vi "AvisoSectorConvert.vi"(7 "output cluster":T1={"Axis scaling Params"={"X right"=0.0, "X left"=0.0, "Y low"=0.0, "Y high"=0.0}, "x scaled"=[], "y scaled"=[], "scales"={"inc x (mm)"=0.0, "inc y (mm)"=0.0}, [], "pixels in x"=256, "pixels in y"=1000}, 10 "Log Lookup":sgl[](array[numeric]), 11 "Raw In":dbl[][](array[numeric])) -> (3 "Sector out":dbl[][](array[numeric]))   [LabVIEW 2022 SP3]
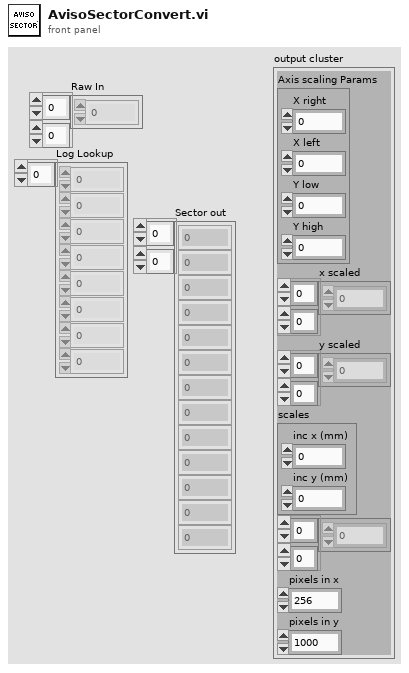
[diagram p1: front panel]
types:
  T1 = cluster{"Axis scaling Params":cluster{"X right":dbl, "X left":dbl, "Y low":dbl, "Y high":dbl}, "x scaled":dbl[][], "y scaled":dbl[][], "scales":cluster{"inc x (mm)":dbl, "inc y (mm)":dbl}, dbl[][], "pixels in x":i16, "pixels in y":i16}
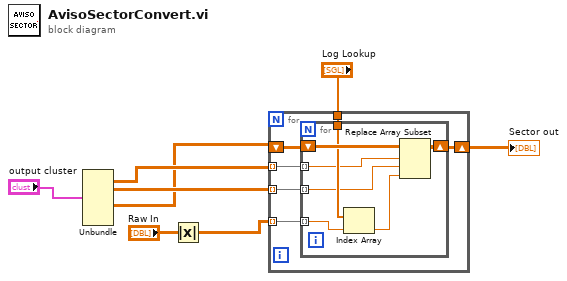
[diagram p0: block diagram]
diagram:
  n1 = Unbundle("output cluster") -> ("x scaled"=w5:dbl[][], "y scaled"=w6:dbl[][], w3:dbl[][])  [unwired: 4 out]
  n2 = Absolute Value(x="Raw In") -> (abs(x)=w4:dbl[][])
  n3 = for {
    tunnel: w4 -> [w14] mode=indexing
    shift-right: [w12] -> w1
    shift-left: w3 -> [w13]
    tunnel: w5 -> [w11] mode=indexing
    tunnel: w6 -> [w10] mode=indexing
    tunnel: "Log Lookup" -> [w9]
    n4 = for {
      tunnel: w14 -> [w19] mode=indexing
      shift-right: [w20] -> w12
      shift-left: w13 -> [w21]
      tunnel: w11 -> [w16] mode=indexing
      tunnel: w10 -> [w15] mode=indexing
      tunnel: w9 -> [w17]
      n5 = Index Array(array=w17, index=w19) -> (element=w18:sgl)
      n6 = Replace Array Subset(array=w21, new element=w18, index (row)=w16, index (col)=w15) -> (w20:dbl[][])
    }
  }
  "Sector out" <- w1
